vi "Sub Initialize.vi"(8 "error in (no error)":errorcluster, 11 "Spectrum Recorder in":refnum<class "Spectrum Recorder.lvclass">) -> (0 "error out":errorcluster, 2 "Initialize Result":refnum<class "Acquired Result.lvclass">, 3 "Spectrum Recorder out":refnum<class "Spectrum Recorder.lvclass">)   [LabVIEW 2016, in "Spectrum Recorder.lvclass"]
uses:
  Spectrum Recorder.lvclass
  C:/github/Measure_core/Worker/Worker.lvclass
  C:/github/Measure_core/Instrument Actor/Instrument Actor.lvclass
  Measure_core/Results/Acquired Result/Acquired Result.lvclass
  Measure_core/Worker/Worker.lvclass/Worker.ctl
  NHMFL_Core/Libraries/Red Pitaya/RP Core/RP Transceiver/Receiver format.ctl
  Spectrum Recorder.lvclass/Spectrum Recorder.ctl
  NHMFL_Core/Libraries/Red Pitaya/RP Core/RP Transceiver/RP Transceiver.lvclass/RP Transceiver.ctl
  NHMFL_Core/Libraries/Red Pitaya/RP Core/RP Instrument/RP Instrument.lvclass/RP Instrument.ctl
  Measure_core/Template Module/Write Active.vi
  NHMFL_Core/Libraries/Red Pitaya/RP Core/RP Transceiver/Write Receiver format.vi
  NHMFL_Core/Libraries/Red Pitaya/RP Core/RP Instrument/Write DDS delay.vi
  Measure_core/Template Module/Read Active.vi
  NHMFL_Core/Libraries/Red Pitaya/RP Core/RP Transceiver/RP Transceiver.lvclass
  C:/github/NHMFL_Core/Libraries/Red Pitaya/RP Core/RP Instrument/RP Instrument.lvclass
  Read Spectrum Recorder Configuration.vi
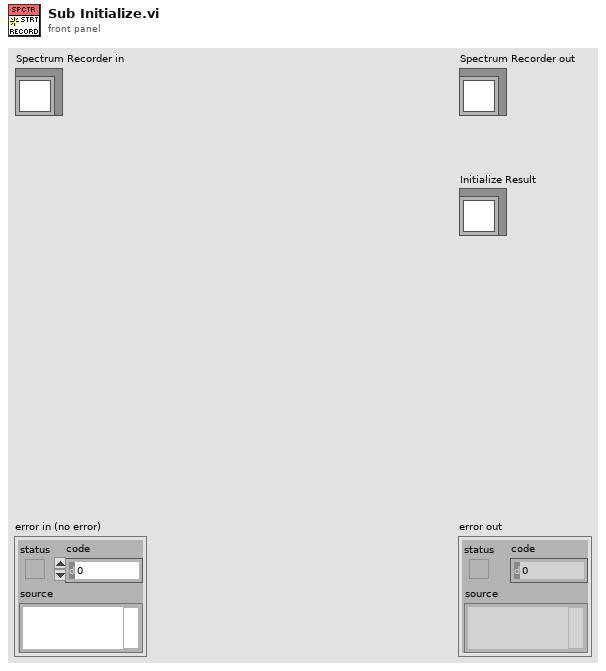
[diagram p1: front panel]
types:
  T1 = typedef "Receiver format.ctl" = enum16{"X-Y-F", "F-X-Y", "X-Y", "X"}
  T2 = typedef "Spectrum Recorder Configuration.ctl" = cluster{"Start":dbl, "End":dbl, "Duration":dbl, "Filter time constant":dbl, "Repeat (-1: forever)":i32, "Update rate":dbl, "Data storage folder":path}
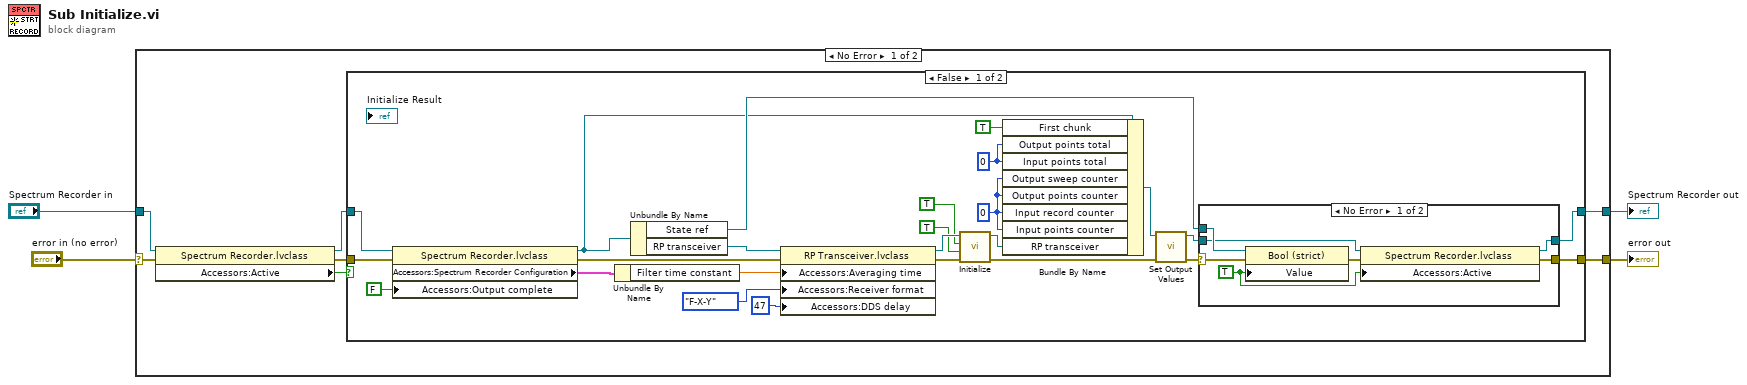
[diagram p0: block diagram]
diagram:
  n1 = case shown="No Error" "error in (no error)" {
    selector: "error in (no error)" -> [w6 w49]
    tunnel: [w9 w49] -> w3
    tunnel: [w11 w48] -> w1
    tunnel: "Spectrum Recorder in" -> [w10 w48]
    frame No Error {
      n2 = property class="Spectrum Recorder.lvclass"(reference=w10, error in=w6) -> (reference out=w8:refnum<class "Spectrum Recorder.lvclass">, error out=w5:errorcluster, "Accessors:Active"=w7:bool)
      n3 = case shown="False" w7 {
        tunnel: w8 -> [w18 w47]
        tunnel: [w20 w47] -> w11
        tunnel: w5 -> [w14 w46]
        tunnel: [w27 w46] -> w9
        frame False {
          w19 = i64 0 ("Output points total")
          w25 = 0 ("Output sweep counter")
          n4 = property class="Spectrum Recorder.lvclass"(reference=w18, error in=w14, "Accessors:Output complete"=FALSE ("Output complete")) -> (reference out=w17:refnum<class "Spectrum Recorder.lvclass">, error out=w13:errorcluster, "Accessors:Spectrum Recorder Configuration"=w16:T2)
          n5 = Unbundle By Name(w16) -> ("Filter time constant"=w15:dbl)
          n6 = Unbundle By Name(w17) -> ("State ref"=w26:refnum<vi>, "RP transceiver"=w29:refnum<class "RP Transceiver.lvclass">)
          n7 = property class="RP Transceiver.lvclass"(reference=w29, error in=w13, "Accessors:Averaging time"=w15, "Accessors:Receiver format"=Receiver_format."F-X-Y" ("Receiver format"), "Accessors:DDS delay"=u32 47 ("DDS delay")) -> (reference out=w34:refnum<class "RP Transceiver.lvclass">, error out=w33:errorcluster)
          n8 = call-dynamic "Initialize.vi"("error in (no error)"=w33, "Send \"Connect client\""=TRUE ("Send \"Connect client\""), "Reset"=TRUE, "RP Transceiver in"=w34) -> ("error out"=w30:errorcluster, "RP Transceiver out"=w23:refnum<class "RP Transceiver.lvclass">)  [unwired: 6 in]
          n9 = Bundle By Name(cluster=w17, "First chunk"=TRUE, "Output points total"=w19, "Input points total"=w19, "Output sweep counter"=w25, "Output points counter"=w25, "Input record counter"=w25, "Input points counter"=w25, "RP transceiver"=w23) -> (w28:refnum<class "Spectrum Recorder.lvclass">)
          n10 = call-dynamic "Set Output Values.vi"("error in (no error)"=w30, "Spectrum Recorder in"=w28) -> ("error out"=w22:errorcluster, "Spectrum Recorder out"=w21:refnum<class "Spectrum Recorder.lvclass">)  [unwired: 8 in]
          n11 = case shown="No Error" w22 {
            selector: w22 -> [w42 w44]
            tunnel: [w37 w44] -> w27
            tunnel: w26 -> [w43 _]
            tunnel: w21 -> [w41 w45]
            tunnel: [w40 w45] -> w20
            frame No Error {
              w39 = TRUE ("Value")
              n12 = property class="Bool (strict)"(reference=w43, error in=w42, "Value"=w39) -> (error out=w38:errorcluster)  [unwired: 1 out]
              n13 = property class="Spectrum Recorder.lvclass"(reference=w41, error in=w38, "Accessors:Active"=w39) -> (reference out=w40:refnum<class "Spectrum Recorder.lvclass">, error out=w37:errorcluster)
            }
            frame Error {
            }
          }
        }
        frame True {
        }
      }
    }
    frame Error {
    }
  }
  "error out" <- w3
  "Spectrum Recorder out" <- w1
